vi "temp.vi"() -> ()   [LabVIEW 2017]
panel:
  out "High Temperature":bool
  out "Low Temperature":bool
  out "Thermometer":dbl(slide) scale=0.0..100.0
  out "Temperatue (C)":dbl
  out "Temperature in (mV)":dbl
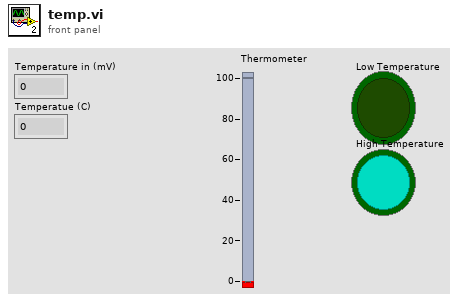
[diagram p1: front panel]
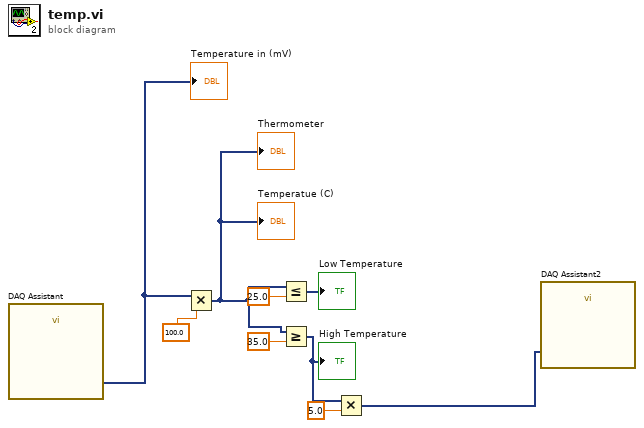
[diagram p0: block diagram]
diagram:
  n1 = call "DAQ Assistant"() -> ("data"=w9:dynamicdata)  [unwired: 16 in, 3 out]
  "Temperature in (mV)" <- w9
  n2 = Multiply(x=w9, y=100.0) -> (x*y=w1:dynamicdata)
  "Temperatue (C)" <- w1
  "Thermometer" <- w1
  n3 = Less Or Equal?(x=w1, y=25.0) -> (x <= y?=→"Low Temperature":dynamicdata)
  n4 = Greater Or Equal?(x=w1, y=35.0) -> (x >= y?=w4:dynamicdata)
  "High Temperature" <- w4
  n5 = Multiply(x=w4, y=5.0) -> (x*y=w2:dynamicdata)
  n6 = call "DAQ Assistant2"("data"=w2) -> ()  [unwired: 16 in, 3 out]
